vi "Init Base Graph.vi"(6 "Z Scale.Marker Values[]":cluster{"Numeric":dbl, "Numeric":u32}[](array[cluster]), 8 "error in (no error)":errorcluster, 9 "Sizes":cluster{"Height":u32, "Width":u32}, 10 "IntGraph Ref":refnum<vi>, 11 "TG Base Graph in":refnum<class "Base Graph.lvclass">) -> (0 "error out":errorcluster, 3 "TG Base Graph out":refnum<class "Base Graph.lvclass">)   [LabVIEW 2023, in "Base Graph.lvclass"]
uses:
  Base Graph.lvclass
  Base Graph.lvclass/Base Graph.ctl
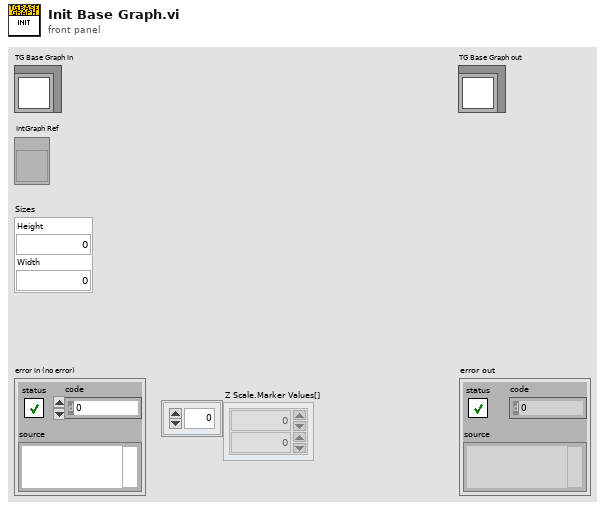
[diagram p1: front panel]
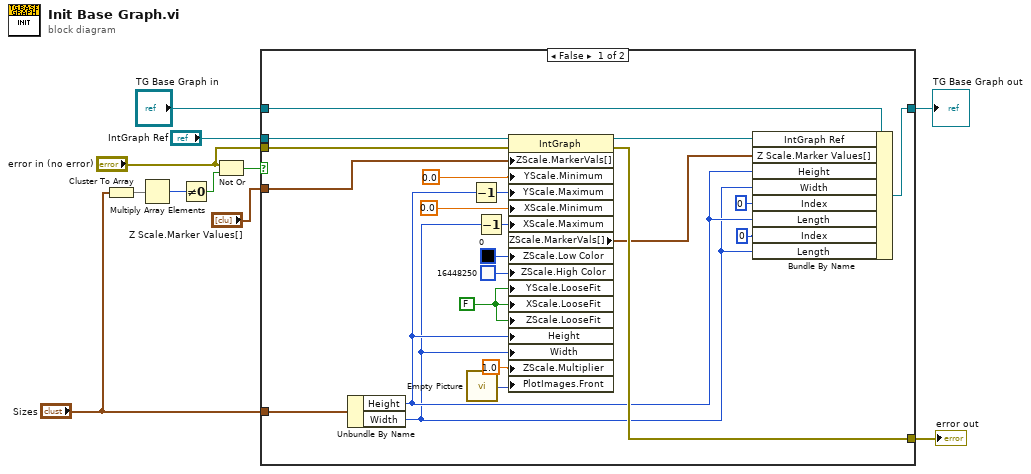
[diagram p0: block diagram]
diagram:
  n1 = Cluster To Array(cluster="Sizes") -> (array=w4:u32[])
  n2 = Multiply Array Elements(1:w4) -> (0:w3:u32)
  n3 = Not Equal To 0?(x=w3) -> (x != 0?=w2:bool)
  n4 = Not Or(1:w2, 2:"error in (no error)") -> (0:w5:bool)
  n5 = case shown="False" w5 {
    tunnel: [w27 w34] -> w11
    tunnel: [w32 w35] -> w9
    tunnel: "TG Base Graph in" -> [w33 w35]
    tunnel: "IntGraph Ref" -> [w31 _]
    tunnel: "Z Scale.Marker Values[]" -> [w29 _]
    tunnel: "Sizes" -> [w28 _]
    tunnel: "error in (no error)" -> [w16 w34]
    frame False {
      w19 = FALSE ("X Scale.Loose Fit")
      n6 = Unbundle By Name(w28) -> ("Height"=w18:u32, "Width"=w17:u32)
      n7 = call "Empty Picture"() -> ("empty picture"=w12:picture)
      n8 = Decrement(x=w18) -> (x-1=w15:u32)
      n9 = Decrement(x=w17) -> (x-1=w14:u32)
      n10 = property class="IntGraph"(reference=w31, error in=w16, "ZScale.MarkerVals[]"=w29, "YScale.Minimum"=0.0 ("Y Scale.Range:Minimum"), "YScale.Maximum"=w15, "XScale.Minimum"=0.0 ("X Scale.Range:Minimum"), "XScale.Maximum"=w14, "ZScale.Low Color"=u32 0 ("Z Scale.Low Color"), "ZScale.High Color"=u32 16448250 ("Z Scale.High Color"), "YScale.LooseFit"=w19, "XScale.LooseFit"=w19, "ZScale.LooseFit"=w19, "Height"=w18, "Width"=w17, "ZScale.Multiplier"=1.0 ("Z Scale.Offset and Multiplier:Multiplier"), "PlotImages.Front"=w12) -> (reference out=w30:refnum<vi>, error out=w27:errorcluster, "ZScale.MarkerVals[]"=w24:cluster{dbl, u32}[])
      n11 = Bundle By Name(cluster=w33, "IntGraph Ref"=w30, "Z Scale.Marker Values[]"=w24, "Height"=w18, "Width"=w17, "Index"=u32 0 ("ROI XY.ROI Y.Index"), "Length"=w18, "Index"=u32 0 ("ROI XY.ROI X.Index"), "Length"=w17) -> (w32:refnum<class "Base Graph.lvclass">)
    }
    frame True {
    }
  }
  "error out" <- w11
  "TG Base Graph out" <- w9
